vi "Controller Test Bench (13).vi"() -> ()   [LabVIEW 2022 SP3]
uses:
  WhiteNoise.ctl
  <vilib>/sound2/lvsound2.llb/Sound Data Format.ctl
  <vilib>/Utility/error.llb/DialogType.ctl
  <vilib>/sound2/lvsound2.llb/Sampling Mode.ctl
  <vilib>/Analysis/3filter.llb/Filter Passband Type.ctl
  <vilib>/Analysis/4window.llb/windowTd.ctl
  <vilib>/DAQmx/read.llb/DAQmx Read (Analog 1D Wfm NChan NSamp).vi
  <vilib>/addons/control/pid/pid.llb/PID Advanced (DBL Array).vi
  <vilib>/addons/control/pid/pid.llb/PID Parameter Manager (DBL Array).vi
  <vilib>/addons/control/pid/pid.llb/PID Derivative Action Buffered (DBL Array).vi
  <vilib>/addons/control/pid/pid.llb/PID Get Advanced Error (DBL Array).vi
  <vilib>/addons/control/pid/pid.llb/PID Integral Action Buffered (DBL Array).vi
  <vilib>/addons/control/pid/pid.llb/PID Resize 1D Array.vi
  <vilib>/addons/control/pid/pid.llb/PID Get Advanced Error (DBL).vi
  <vilib>/DAQmx/create/channels.llb/DAQmx Create Channel (AI-Acceleration-Accelerometer).vi
  <vilib>/DAQmx/configure/timing.llb/DAQmx Timing (Sample Clock).vi
  <vilib>/DAQmx/configure/task.llb/DAQmx Configure Logging (TDMS).vi
  <vilib>/sound2/lvsound2.llb/Sound Output Set Volume (Single).vi
  <vilib>/DAQmx/create/channels.llb/DAQmx Create Channel (AO-Voltage-Basic).vi
  <vilib>/Analysis/3filter.llb/Butterworth Filter (DBL).vi
  <vilib>/sound2/lvsound2.llb/Sound Output Write (DBL Single).vi
  <vilib>/DAQmx/miscellaneous.llb/DAQmx Fill In Error Info.vi
  <vilib>/measure/maspectr.llb/FFT Spectrum (Mag-Phase) for N Chan.vi
  <vilib>/measure/NI_MAPro.lvlib
  <resource>/objmgr/daqmx.rc
  <vilib>/Analysis/NI_AALPro.lvlib
  <vilib>/measure/NI_MABase.lvlib
  <vilib>/addons/control/pid/NI_PID_pid.lvlib
  <vilib>/Analysis/NI_AALBase.lvlib
  <vilib>/DAQmx/write.llb/DAQmx Write (Analog 1D DBL 1Chan NSamp).vi
panel:
  in  "Sample Rate":dbl=1024.0
  in  "Raw Data":bool
  in  "Active Control":bool
  out "Waveform Graph":waveform(dbl)(graph)
  in  "Folder to save file to":path=path "C:/Users/LAV-UFSC-2023/Documents/LAV-TCC/Dados-Experimentos/Dados-Bancada-LABVIEW"
  in  "Time Out (s)":dbl=60.0
  out "Active Controller Output":dbl[](graph)
  out "Elapsed Time":i32 caption="Elapsed Time (s)" format="%.2f"
  out "Accel.1":waveform(dbl)[](graph)
  in  "Output Noise":bool=TRUE
  in  "?":enum32{"White Noise", "Harmonic"}(tab)=enum."Harmonic"
  in  "Cluster":T2={"Seed"=0.0, "Standard Deviation"=1.0, "Reset"=TRUE, "Iterator"=1.0, "Lower Cut-Off 2"=5.0, "Upper Cut-Off 2"=350.0} {"Upper Cut-Off 2" min=5.0 max=350.0 step=10.0; "Lower Cut-Off 2" min=5.0 max=350.0 step=10.0; "Standard Deviation" min=0.001 max=3.5 step=0.05 format="%0.2p"}
  in  "Cluster 2":T3={"Waveform Type"=0, "Frequency"=10.0, "Amplitude"=0.25} {"Frequency" min=5.0 max=350.0 step=10.0 format="%0.2p"; "Waveform Type" items=["Sine Wave", "Triangle Wave", "Square Wave", "Sawtooth Wave"]; "Amplitude" min=0.001 max=0.3 step=0.05 format="%0.2p"}
  in  "Fs":dbl=16384.0
  in  "#s":dbl=360.0
  in  "Tab Control":T4(tab)
  in  "setpoint":dbl[](array[numeric])=[0.0] format="%.2f"
  in  "PID gains":T5(array[cluster])=[{"proportional gain (Kc)"=1.0, "integral time (Ti, min)"=0.01, "derivative time (Td, min)"=0.0}] {"derivative time (Td, min)" format="%.3f"; "integral time (Ti, min)" format="%.3f"; "proportional gain (Kc)" step=0.01 format="%.3f"}
  in  "output range":cluster{"output high":dbl, "output low":dbl}[](array[cluster])=[{"output high"=100.0, "output low"=-100.0}] {"output low" format="%.2f"; "output high" format="%.2f"}
  in  "manual control":dbl[](array[numeric])=[0.0] format="%.2f"
  in  "setpoint range":T6(array[cluster])=[{"setpoint high"=100.0, "setpoint low"=0.0}] {"setpoint high" format="%.2f"; "setpoint low" format="%.2f"}
  in  "Setpoint":dbl
  in  "Gain":dbl min=0.0 step=0.01
  in  "Upper Cut-Off":dbl=400.0
  in  "Lower Cut-Off":dbl=100.0
  out "Phase 2":cluster{"f0":dbl, "df":dbl, "phase":dbl[]}[](graph)
  out "Mag 2":cluster{"f0":dbl, "df":dbl, "magnitude":dbl[]}[](graph)
  in  "FFT":bool=TRUE
  in  "FFT":bool
  in  "Raw Data":bool=TRUE
  # "Data Acquisition"
  # "Log"
  # "Read"
  # "Output"
  # "Filter"
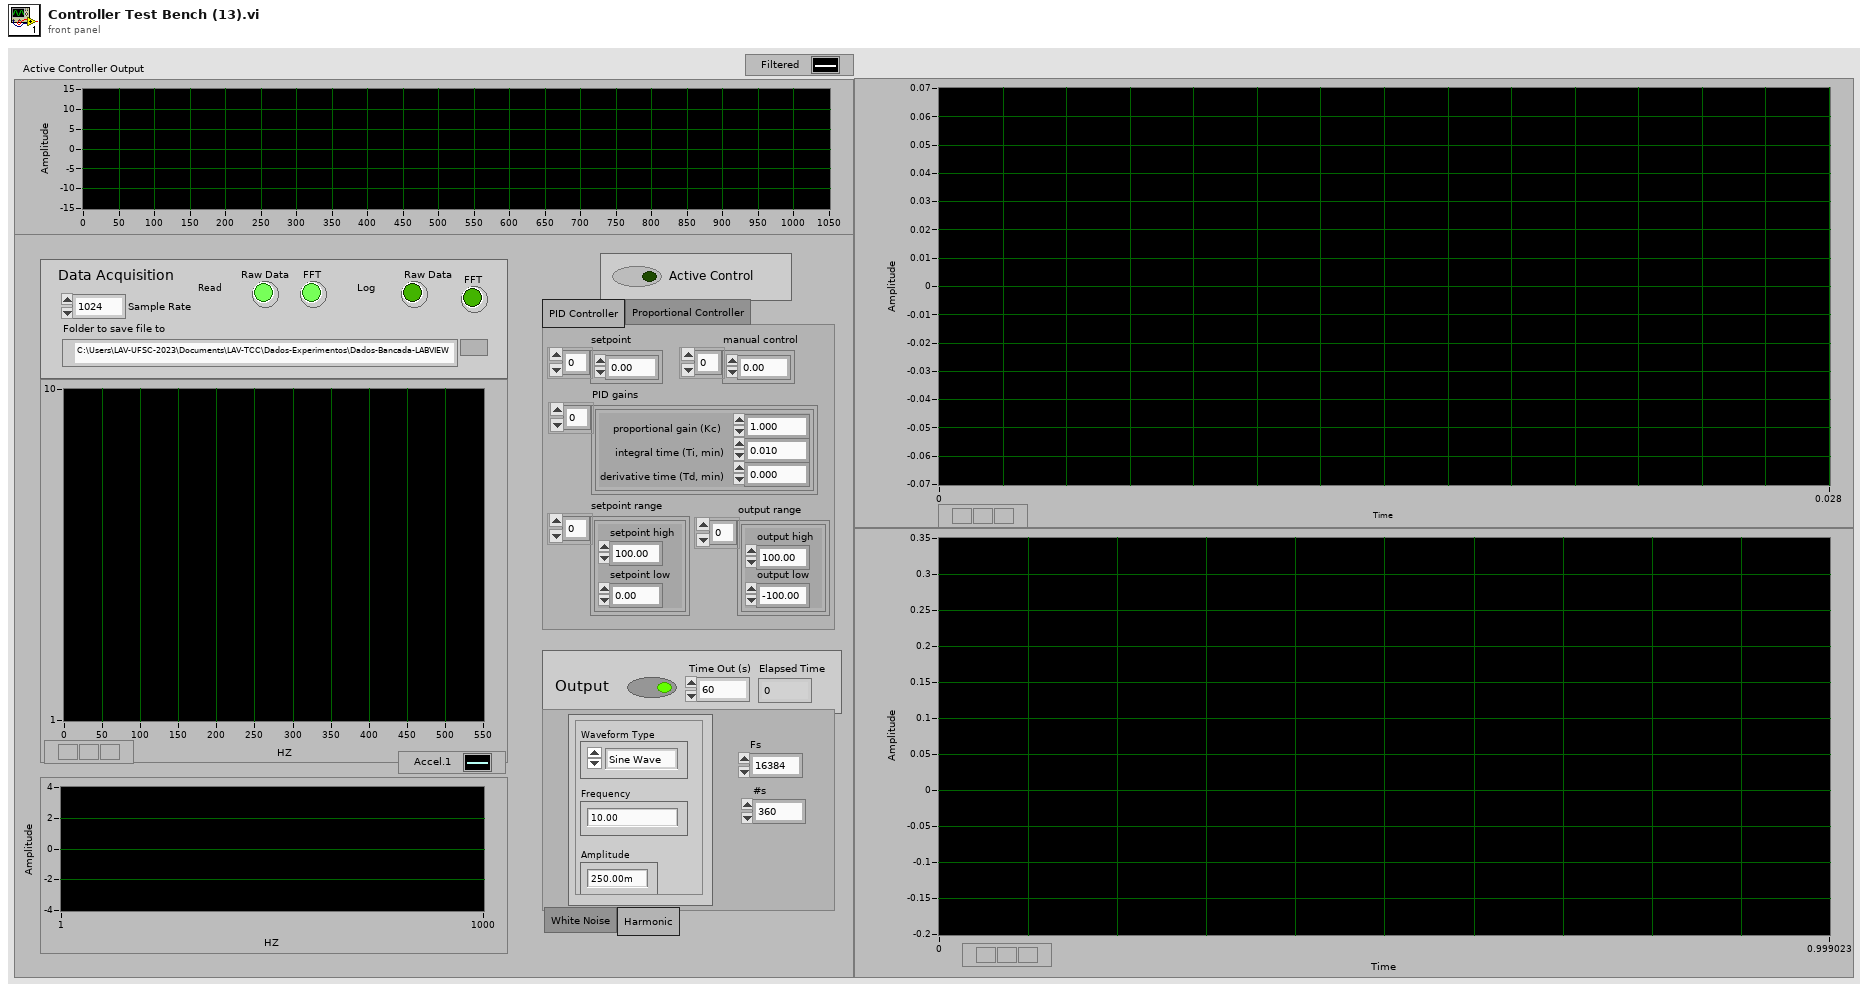
[diagram p1: front panel]
types:
  T1 = typedef "WhiteNoise.ctl" = dbl
  T2 = cluster{"Seed":T1, "Standard Deviation":dbl, "Reset":bool, "Iterator":dbl, "Lower Cut-Off 2":dbl, "Upper Cut-Off 2":dbl}
  T3 = cluster{"Waveform Type":u16, "Frequency":dbl, "Amplitude":dbl}
  T4 = enum32{"PID Controller", "Proportional Controller"}
  T5 = cluster{"proportional gain (Kc)":dbl, "integral time (Ti, min)":dbl, "derivative time (Td, min)":dbl}[]
  T6 = cluster{"setpoint high":dbl, "setpoint low":dbl}[]
  T7 = typedef "Sampling Mode.ctl" = i32
  T8 = typedef "DialogType.ctl" = u16
  T9 = typedef "Sound Data Format.ctl" = cluster{"sample rate (S/s)":dbl, "number of channels":i32, "bits per sample":i32}
  T10 = typedef "Sound Output Task ID.ctl" = u32
  T11 = typedef "NI_AALBase.lvlib/Filter Passband Type.ctl" = enum32{"Lowpass", "Highpass", "Bandpass", "Bandstop"}
  T12 = cluster{"dB On (F)":bool, "unwrap phase (F)":bool, "convert to degree (F)":bool}
  T13 = cluster{"averaging mode":enum16{"No averaging", "Vector averaging", "RMS averaging", "Peak hold"}, "weighting mode":enum16{"Linear", "Exponential"}, "number of averages":u32}
  T14 = typedef "NI_AALPro.lvlib/windowTd.ctl" = u32
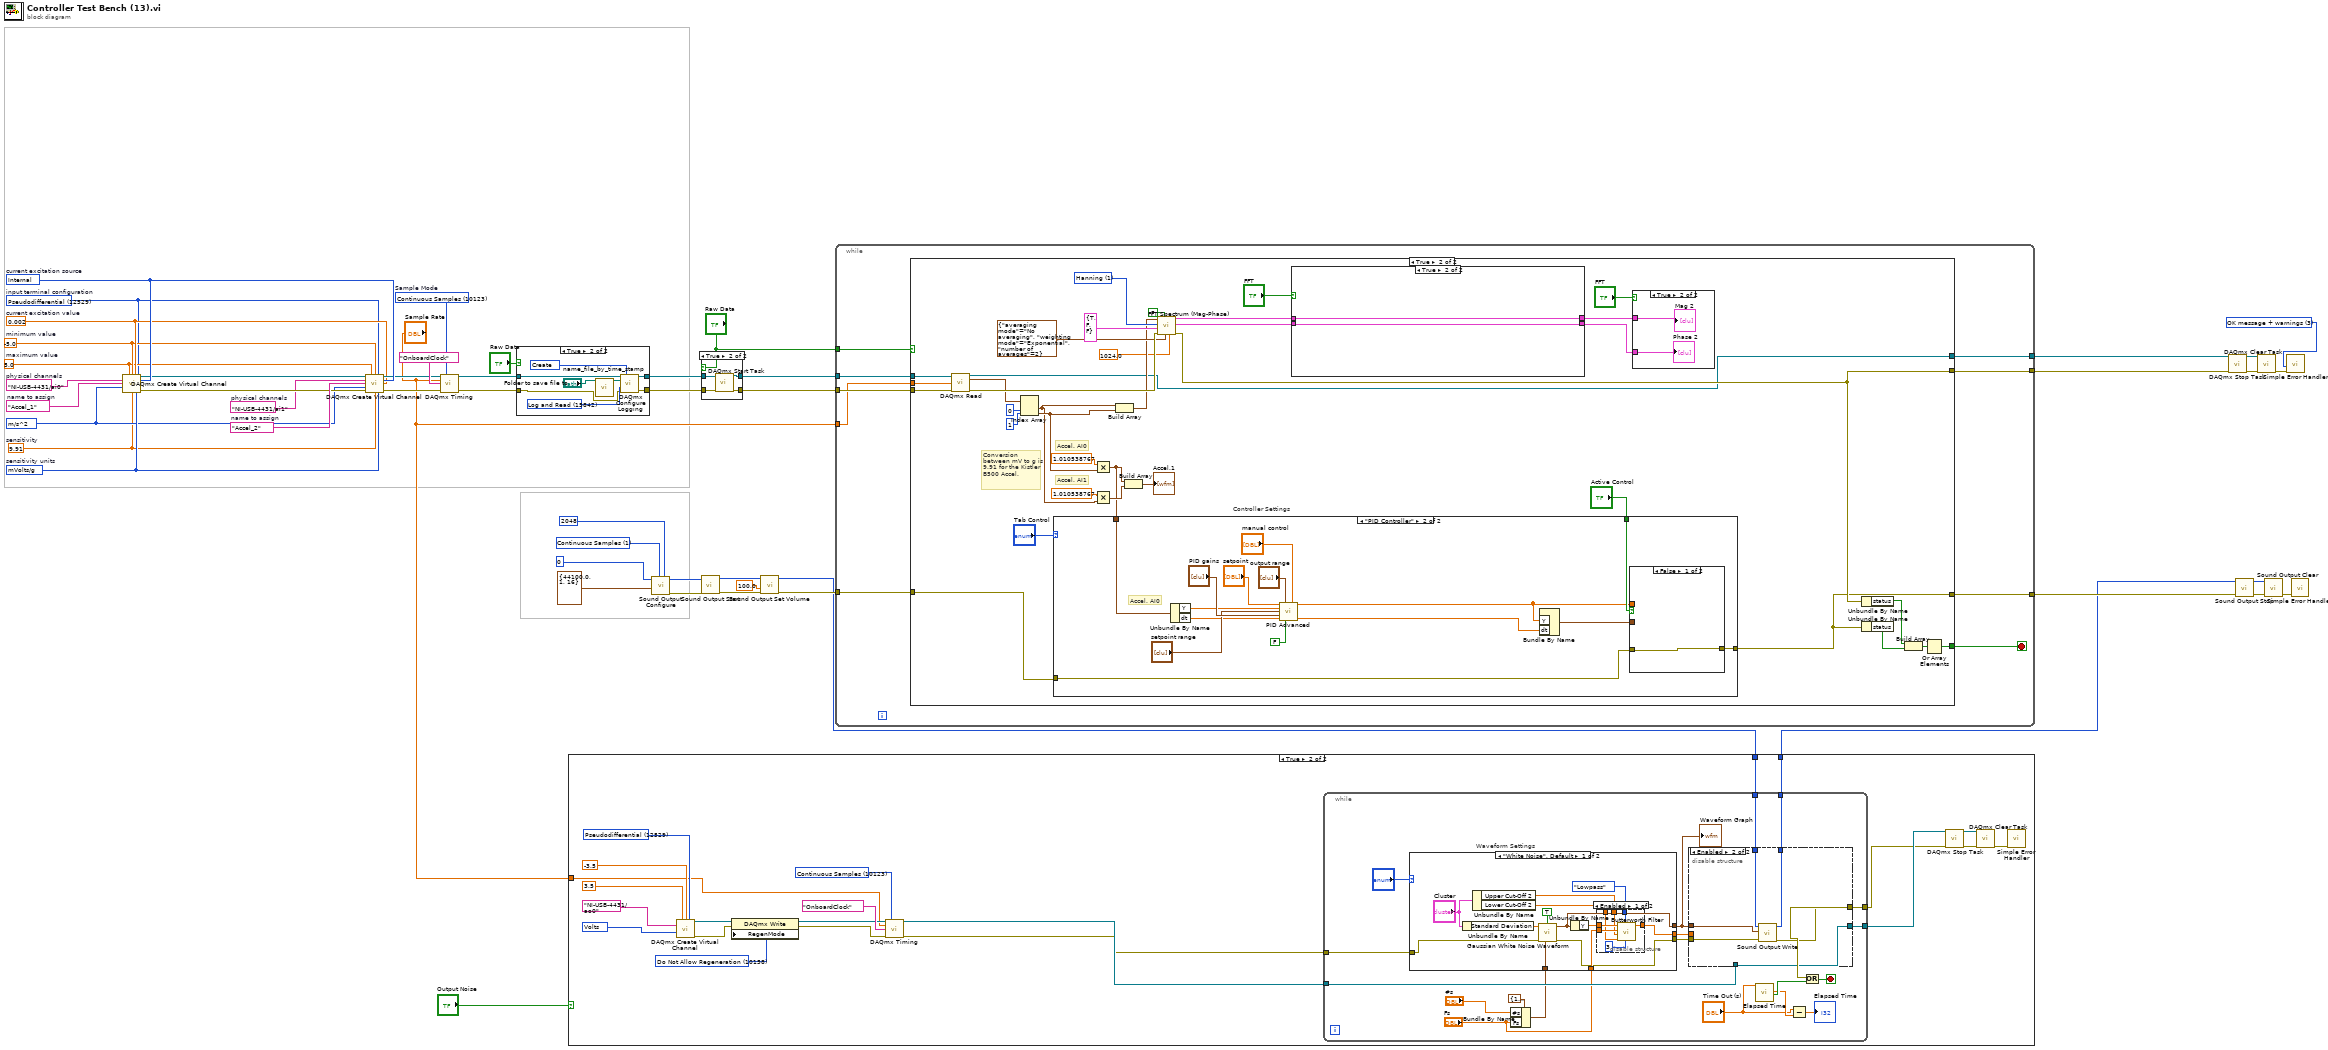
[diagram p0: block diagram]
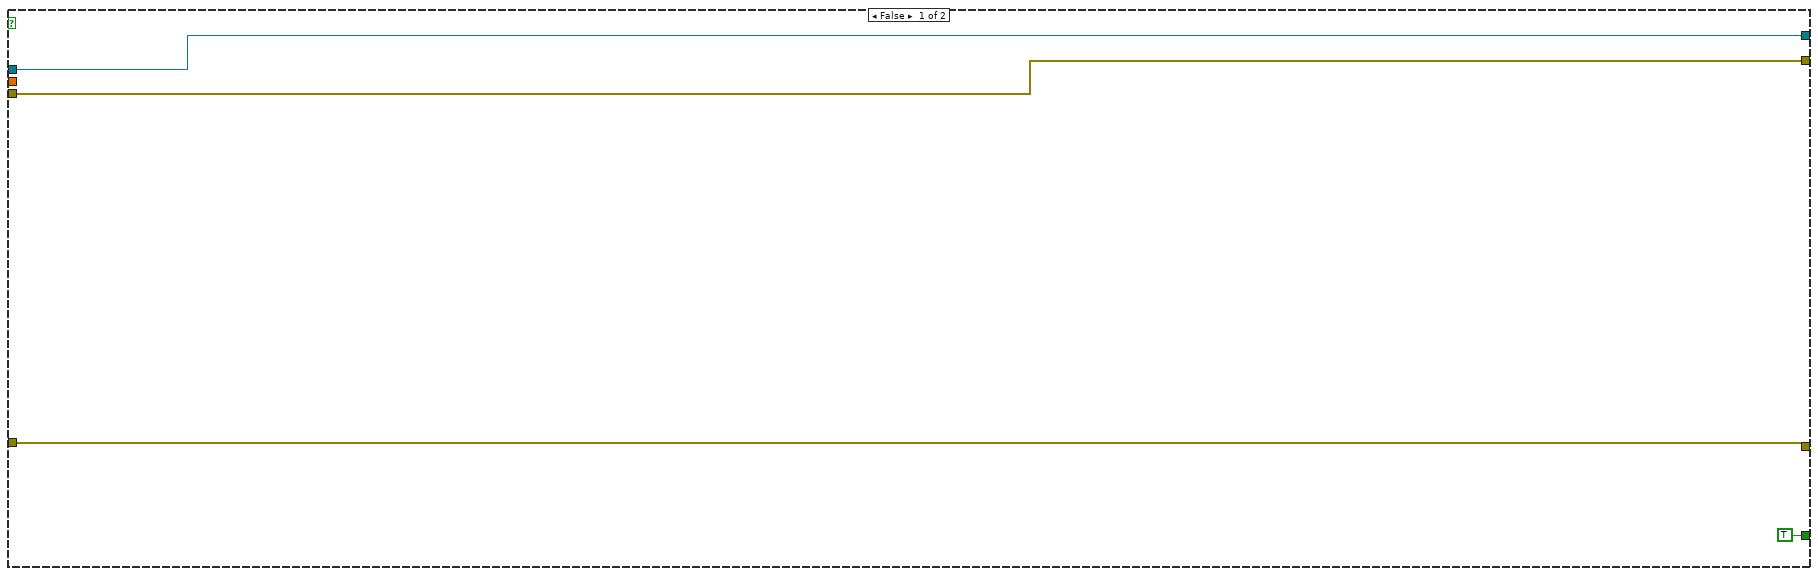
[diagram p2: hidden frame]
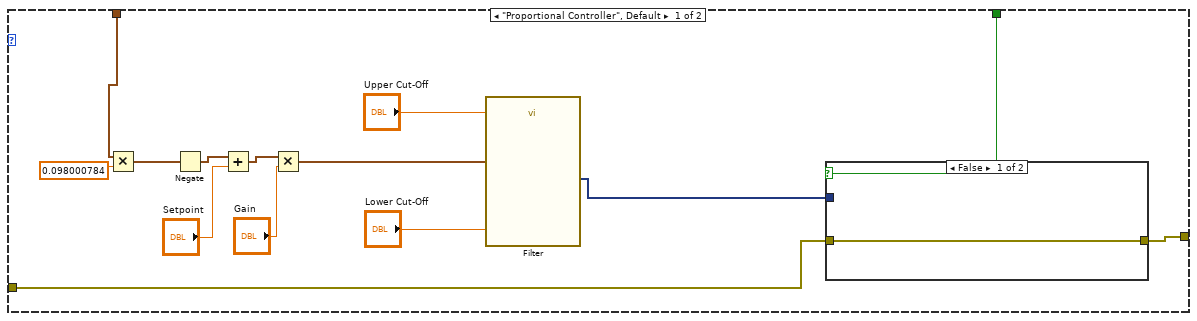
[diagram p3: hidden frame]
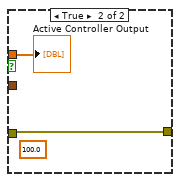
[diagram p5: hidden frame]
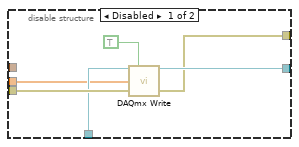
[diagram p10: hidden frame]
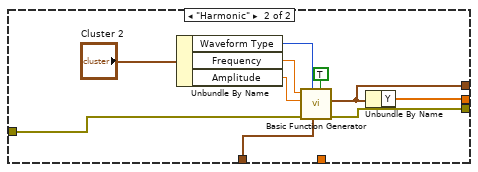
[diagram p12: hidden frame]
diagram:
  w14 = 12470 items=["g"=10186, "m/s^2"=12470, "in/s^2"=12471, "From Custom Scale"=10065] ("units")
  w15 = 12509 items=["mVolts/g"=12509, "Volts/g"=12510]  # sensitivity units
  w13 = 9.91  # sensitivity
  w33 = 0.002  # current excitation value
  w36 = 10200 items=["Internal"=10200, "External"=10167, "None"=10230]  # current excitation source
  w28 = tag "NI-USB-4431/ai0"  # physical channels
  w40 = 10123 items=["Finite Samples"=10178, "Continuous Samples"=10123, "Hardware Timed Single Point"=12522]  # Sample Mode
  w30 = 12529 items=["default"=-1, "RSE"=10083, "NRSE"=10078, "Differential"=10106, "Pseudodifferential"=12529]  # input terminal configuration
  w32 = -5.0  # minimum value
  w31 = 5.0  # maximum value
  w41 = "Accel_1"  # name to assign
  w29 = tag "NI-USB-4431/ai1"  # physical channels
  w38 = "Accel_2"  # name to assign
  w42 = T7 1 items=["Finite Samples", "Continuous Samples"] ("sample mode")
  w43 = T8 3 items=["no dialog", "OK message", "continue or stop message", "OK message + warnings", "continue/stop + warnings"] ("type of dialog (OK msg:1)")
  n1 = call-poly <vilib>:"DAQmx Create Virtual Channel.vi"("maximum value"=w31, "minimum value"=w32, "input terminal configuration"=w30, "physical channels"=w28, "current excitation source"=w36, "name to assign"=w41, "current excitation value"=w33, "units"=w14, "sensitivity"=w13, "sensitivity units"=w15) -> ("task out"=w16:refnum<k21>, "error out"=w37:errorcluster)  [unwired: 4 in]
  n2 = call-poly <vilib>:"DAQmx Create Virtual Channel.vi"("task in"=w16, "maximum value"=w31, "minimum value"=w32, "input terminal configuration"=w30, "physical channels"=w29, "current excitation source"=w36, "name to assign"=w38, "current excitation value"=w33, "units"=w14, "error in"=w37, "sensitivity"=w13, "sensitivity units"=w15) -> ("task out"=w35:refnum<k21>, "error out"=w34:errorcluster)  [unwired: 2 in]
  n3 = call-poly <vilib>:"DAQmx Timing.vi"("task/channels in"=w35, "sample mode"=w40, "rate"="Sample Rate", "source"=tag "OnboardClock" ("Sample Clock Source"), "error in"=w34) -> ("task out"=w12:refnum<k21>, "error out"=w9:errorcluster)  [unwired: 9 in]
  n4 = case shown="True" "Raw Data" {
    tunnel: w12 -> [w52 w57]
    tunnel: [w52 w58] -> w11
    tunnel: [w51 w54] -> w10
    tunnel: w9 -> [w51 w53]
    frame False {
    }
    frame True {
      w59 = 15848 items=["Open"=10437, "Open or Create"=15846, "Create or Replace"=15847, "Create"=15848] ("operation")
      w60 = 15842 items=["Off"=10231, "Log"=15844, "Log and Read"=15842] ("logging mode")
      n5 = call "name_file_by_time_stamp.vi"("Folder to save file to"="Folder to save file to") -> ("New file path"=w56:path)  [unwired: 10 in]
      n6 = call-poly <vilib>:"DAQmx Configure Logging.vi"("task/channels in"=w57, "operation"=w59, "file path"=w56, "logging mode"=w60, "error in"=w53) -> ("task out"=w58:refnum<k21>, "error out"=w54:errorcluster)  [unwired: 9 in]
    }
  }
  n7 = call <vilib>:"Sound Output Configure.vi"("number of samples/ch"=2048 ("Number of Samples/ch"), "sample mode"=w42, "sound format"=T9 {"sample rate (S/s)"=44100.0, "number of channels"=1, "bits per sample"=16} ("Sound Format"), "device ID"=u32 0 ("Device ID")) -> ("error out"=w24:errorcluster, "task ID"=w23:T10)  [unwired: 6 in]
  n8 = case shown="True" "Raw Data" {
    tunnel: w10 -> [w61 w66]
    tunnel: w11 -> [w62 w65]
    tunnel: [w62 w64] -> w20
    tunnel: [w61 w63] -> w21
    frame False {
    }
    frame True {
      n9 = call <vilib>:"DAQmx Start Task.vi"("task/channels in"=w65, "error in"=w66) -> ("task out"=w64:refnum<k21>, "error out"=w63:errorcluster)  [unwired: 12 in]
    }
  }
  n10 = call <vilib>:"Sound Output Start.vi"("error in (no error)"=w24, "task ID"=w23) -> ("error out"=w5:errorcluster, "task ID out"=w4:T10)  [unwired: 8 in]
  n11 = call-poly <vilib>:"Sound Output Set Volume.vi"("error in (no error)"=w5, "volume"=100.0, "task ID"=w4) -> ("error out"=w3:errorcluster, "task ID out"=w1:T10)  [unwired: 7 in]
  n12 = case shown="True" "Output Noise" {
    tunnel: "Sample Rate" -> [_ w71]
    tunnel: [w67 w69] -> w2
    tunnel: w1 -> [w67 w68]
    frame False {
    }
    frame True {
      w78 = 10123 items=["Finite Samples"=10178, "Continuous Samples"=10123, "Hardware Timed Single Point"=12522] ("sample mode")
      w82 = 10158 items=["Allow Regeneration"=10097, "Do Not Allow Regeneration"=10158] ("RegenMode")
      w87 = 12529 items=["Default"=-1, "RSE"=10083, "Differential"=10106, "Pseudodifferential"=12529] ("output terminal configuration")
      w85 = 10348 items=["Volts"=10348, "From Custom Scale"=10065] ("units")
      n13 = call-poly <vilib>:"DAQmx Create Virtual Channel.vi"("maximum value"=3.5, "minimum value"=-3.5, "output terminal configuration"=w87, "physical channels"=tag "NI-USB-4431/ao0", "units"=w85) -> ("task out"=w81:refnum<k21>, "error out"=w83:errorcluster)  [unwired: 9 in]
      n14 = property class="DAQmx Write"(reference=w81, error in=w83, "RegenMode"=w82) -> (reference out=w79:refnum<k21>, error out=w80:errorcluster)
      n15 = call-poly <vilib>:"DAQmx Timing.vi"("task/channels in"=w79, "sample mode"=w78, "rate"=w71, "source"=tag "OnboardClock" ("Sample Clock Source"), "error in"=w80) -> ("task out"=w77:refnum<k21>, "error out"=w76:errorcluster)  [unwired: 9 in]
      n16 = while {
        tunnel: [w106] -> w72
        tunnel: w77 -> [w105]
        tunnel: w76 -> [w99]
        tunnel: [w98] -> w70
        tunnel: [w92] -> w69
        tunnel: w68 -> [w91]
        stop <- w104 stop-if-true
        # "Waveform Settings"
        n17 = Bundle By Name(cluster=cluster{"Fs":dbl, "#s":dbl} {"Fs"=1000.0, "#s"=1000.0} ("sampling info"), "#s"="#s", "Fs"="Fs") -> (w96:cluster{"Fs":dbl, "#s":dbl})
        n18 = case shown="\"White Noise\", Default" "?" {
          tunnel: w96 -> [w133 w150]
          tunnel: w99 -> [w132 w151]
          tunnel: [w122 w149] -> w107
          tunnel: [w123 w143] -> w94
          tunnel: "Fs" -> [w126 _]
          tunnel: [w121 w142] -> w90
          frame "White Noise", Default {
            n19 = Unbundle By Name("Cluster") -> ("Standard Deviation"=w129:dbl)
            n20 = Unbundle By Name("Cluster") -> ("Upper Cut-Off 2"=w124:dbl, "Lower Cut-Off 2"=w125:dbl)
            n21 = call <vilib>:"Gaussian White Noise Waveform.vi"("sampling info"=w133, "reset signal"=TRUE, "error in (no error)"=w132, "standard deviation"=w129) -> ("error out"=w122:errorcluster, "signal out"=w121:waveform(dbl))  [unwired: 6 in]
            n22 = Unbundle By Name(w121) -> ("Y"=w127:dbl[])
            n23 = disable-structure shown="Enabled" {
              disable-tunnel: Filter_Passband_Type."Lowpass" ("filter type") -> [w140 _]
              disable-tunnel: w127 -> [w139 w141]
              disable-tunnel: w126 -> [w138 _]
              disable-tunnel: w125 -> [w137 _]
              disable-tunnel: w124 -> [w136 _]
              disable-tunnel: [w134 w141] -> w123
              frame Enabled {
                n24 = call-poly <vilib>:"Butterworth Filter.vi"("order"=3, "filter type"=w140, "low cutoff freq: fl"=w137, "high cutoff freq: fh"=w136, "sampling freq: fs"=w138, "X"=w139) -> ("Filtered X"=w134:dbl[])  [unwired: 2 in, 1 out]
              }
              frame Disabled {
              }
            }
          }
          frame "Harmonic" {
            n25 = Unbundle By Name("Cluster 2") -> ("Waveform Type"=w147:u16, "Frequency"=w146:dbl, "Amplitude"=w145:dbl)
            n26 = call <vilib>:"Basic Function Generator.vi"("reset signal"=TRUE, "sampling info"=w150, "signal type"=w147, "error in (no error)"=w151, "amplitude"=w145, "frequency"=w146) -> ("error out"=w149:errorcluster, "signal out"=w142:waveform(dbl))  [unwired: 3 in, 1 out]
            n27 = Unbundle By Name(w142) -> ("Y"=w143:dbl[])
          }
        }
        "Waveform Graph" <- w90
        n28 = disable-structure shown="Enabled" {
          disable-tunnel: w107 -> [w114 w119]
          disable-tunnel: [w112 w120] -> w106
          disable-tunnel: w105 -> [w111 w120]
          disable-tunnel: [w110 w118] -> w98
          disable-tunnel: w94 -> [w109 _]
          disable-tunnel: w90 -> [_ w115]
          disable-tunnel: [_ w117] -> w92
          disable-tunnel: w91 -> [_ w116]
          frame Disabled {
            n29 = call-poly <vilib>:"DAQmx Write.vi"("task/channels in"=w111, "auto start"=TRUE, "data"=w109, "error in"=w114) -> ("task out"=w112:refnum<k21>, "error out"=w110:errorcluster)  [unwired: 9 in, 1 out]
          }
          frame Enabled {
            n30 = call-poly <vilib>:"Sound Output Write.vi"("error in (no error)"=w119, "data"=w115, "task ID"=w116) -> ("error out"=w118:errorcluster, "task ID out"=w117:T10)  [unwired: 7 in]
          }
        }
        n31 = call "Elapsed Time"("Time Target (s)"="Time Out (s)") -> ("Elapsed Time (s)"=w101:dbl, "Time has Elapsed"=w102:bool)  [unwired: 11 in, 6 out]
        n32 = Subtract(x="Time Out (s)", y=w101) -> (x-y=→"Elapsed Time":dbl)
        n33 = Or(x=w98, y=w102) -> (x .or. y?=w104:bool)
      }
      n34 = call <vilib>:"DAQmx Stop Task.vi"("task/channels in"=w72, "error in"=w70) -> ("task out"=w75:refnum<k21>, "error out"=w74:errorcluster)  [unwired: 12 in]
      n35 = call <vilib>:"DAQmx Clear Task.vi"("task in"=w75, "error in"=w74) -> ("error out"=w73:errorcluster)  [unwired: 13 in]
      n36 = call <vilib>:"Simple Error Handler.vi"("error in (no error)"=w73) -> ()  [unwired: 4 in, 5 out]
    }
  }
  n37 = while {
    tunnel: "Raw Data" -> [w160]
    tunnel: w3 -> [w159]
    tunnel: w21 -> [w158]
    tunnel: w20 -> [w157]
    tunnel: [w156] -> w19
    tunnel: [w155] -> w18
    tunnel: [w154] -> w17
    tunnel: "Sample Rate" -> [w152]
    stop <- w153 stop-if-true
    n38 = case shown="True" w160 {
      tunnel: w157 -> [w164 w200]
      tunnel: w158 -> [w163 w199]
      tunnel: [w164 w175] -> w155
      tunnel: [w163 w188] -> w156
      tunnel: w159 -> [w162 w184]
      tunnel: [w162 w183] -> w154
      tunnel: [TRUE w182] -> w153
      tunnel: w152 -> [_ w166]
      frame False {
      }
      frame True {
        w187 = T14 1 items=["Rectangle"=0, "Hanning"=1, "Hamming"=2, "Blackman-Harris"=3, "Exact Blackman"=4, "Blackman"=5, "Flat Top"=6, "4 Term B-Harris "=7, "7 Term B-Harris"=8, "Low Sidelobe"=9, "Blackman Nuttall"=11, "Triangle"=30, "Bartlett-Hanning"=31, "Bohman"=32, "Parzen"=33, "Welch"=34, "Kaiser"=60, "Dolph-Chebyshev"=61, "Gaussian"=62] ("window")
        # "Accel. AI1"
        # "Accel. AI0"
        # "Conversion between mV to g is 9.91 for the Kistler B500 Accel."
        # "Controller Settings"
        n39 = call-poly <vilib>:"DAQmx Read.vi"("task/channels in"=w200, "number of samples per channel"=w166, "error in"=w199) -> ("task out"=w175:refnum<k21>, "data"=w177:waveform(dbl)[], "error out"=w189:errorcluster)  [unwired: 10 in]
        n40 = Index Array(array=w177, index #1=0 ("index"), index #2=1 ("index")) -> (element #1=w171:waveform(dbl), element #2=w172:waveform(dbl))
        n41 = Multiply(x=1.010538767, y=w172) -> (x*y=w168:waveform(dbl))
        n42 = case shown="\"PID Controller\"" "Tab Control" {
          tunnel: w184 -> [w209 w229]
          tunnel: "Active Control" -> [w208 w228]
          tunnel: [w210 w227] -> w183
          tunnel: w168 -> [w202 w223]
          frame "Proportional Controller", Default {
            n43 = Multiply(x=w202, y=0.098000784) -> (x*y=w204:waveform(dbl))
            n44 = Negate(x=w204) -> (-x=w213:waveform(dbl))
            n45 = Add(x=w213, y="Setpoint") -> (x+y=w212:waveform(dbl))
            n46 = Multiply(x=w212, y="Gain") -> (x*y=w207:waveform(dbl))
            n47 = call "Filter"("Lower Cut-Off"="Lower Cut-Off", "Upper Cut-Off"="Upper Cut-Off", "Signal"=w207) -> ("Filtered Signal"=w201:dynamicdata)  [unwired: 7 in, 1 out]
            n48 = case shown="False" w208 {
              tunnel: w209 -> [w215 w216]
              tunnel: [w215 w216] -> w210
              tunnel: w201 -> [_ _]
              frame False {
              }
              frame True {
              }
            }
          }
          frame "PID Controller" {
            # "Accel. AI0"
            n49 = Unbundle By Name(w223) -> ("Y"=w224:dbl[], "dt"=w220:dbl)
            n50 = call-poly <vilib>:"PID Advanced.vi"("setpoint"="setpoint", "output range"="output range", "manual control"="manual control", "process variable"=w224, "setpoint range"="setpoint range", "PID gains"="PID gains", "dt (s)"=w220, "reinitialize? (F)"=FALSE) -> ("output"=w218:dbl[], "dt out (s)"=w219:dbl)  [unwired: 6 in]
            n51 = Bundle By Name("Y"=w218, "dt"=w219) -> (w217:waveform(dbl))  [unwired: 1 in]
            n52 = case shown="False" w228 {
              tunnel: w229 -> [w232 w233]
              tunnel: [w232 w233] -> w227
              tunnel: w218 -> [_ w234]
              tunnel: w217 -> [_ _]
              frame False {
              }
              frame True {
                (unwired) 100.0 ("volume")
                "Active Controller Output" <- w234
              }
            }
          }
        }
        n53 = Multiply(x=1.010538767, y=w171) -> (x*y=w169:waveform(dbl))
        n54 = Build Array(w171, w172) -> (w176:waveform(dbl)[])
        n55 = Build Array(w168, w169) -> (→"Accel.1":waveform(dbl)[])
        n56 = call-poly <vilib>:"FFT Spectrum (Mag-Phase).vi"("window parameter"=1024.0, "averaging parameters"=T13 {"averaging mode"=enum."No averaging", "weighting mode"=enum."Exponential", "number of averages"=2}, "restart averaging (F)"=FALSE, "error in (no error)"=w189, "view"=T12 {"dB On (F)"=TRUE, "unwrap phase (F)"=FALSE, "convert to degree (F)"=FALSE}, "window"=w187, "time signals"=w176) -> ("error out"=w188:errorcluster, "phases"=w194:cluster{"f0":dbl, "df":dbl, "phase":dbl[]}[], "magnitudes"=w195:cluster{"f0":dbl, "df":dbl, "magnitude":dbl[]}[])  [unwired: 2 out]
        n57 = case shown="True" "FFT" {
          tunnel: w195 -> [w235 w238]
          tunnel: w194 -> [w236 w237]
          tunnel: [w236 w237] -> w193
          tunnel: [w235 w238] -> w192
          frame False {
          }
          frame True {
          }
        }
        n58 = case shown="True" "FFT" {
          tunnel: w192 -> [_ w240]
          tunnel: w193 -> [_ w239]
          frame False {
          }
          frame True {
            "Mag 2" <- w240
            "Phase 2" <- w239
          }
        }
        n59 = Unbundle By Name(w188) -> ("status"=w186:bool)
        n60 = Unbundle By Name(w183) -> ("status"=w191:bool)
        n61 = Build Array(w186, w191) -> (w198:bool[])
        n62 = Or Array Elements(Boolean array=w198) -> (logical OR=w182:bool)
      }
    }
  }
  n63 = call <vilib>:"DAQmx Stop Task.vi"("task/channels in"=w18, "error in"=w19) -> ("task out"=w46:refnum<k21>, "error out"=w45:errorcluster)  [unwired: 12 in]
  n64 = call <vilib>:"Sound Output Stop.vi"("error in (no error)"=w17, "task ID"=w2) -> ("error out"=w27:errorcluster, "task ID out"=w26:T10)  [unwired: 8 in]
  n65 = call <vilib>:"DAQmx Clear Task.vi"("task in"=w46, "error in"=w45) -> ("error out"=w47:errorcluster)  [unwired: 13 in]
  n66 = call <vilib>:"Sound Output Clear.vi"("error in (no error)"=w27, "task ID"=w26) -> ("error out"=w25:errorcluster)  [unwired: 9 in]
  n67 = call <vilib>:"Simple Error Handler.vi"("type of dialog (OK msg:1)"=w43, "error in (no error)"=w47) -> ()  [unwired: 3 in, 5 out]
  n68 = call <vilib>:"Simple Error Handler.vi"("error in (no error)"=w25) -> ()  [unwired: 4 in, 5 out]
